vi "ASIOInfo.vi"() -> ()   [LabVIEW 2016]
uses:
  WaveIO.llb/ASIO_Informations.ctl
panel:
  out "ASIO Device Infos":T1[](array[typedef])
  in  "Direction (Input)":u16(ring)=3 items=["Input", "Output", "Loopback", "ASIO input", "ASIO output"]
  out "Number of Devices":i32=1
  # "ASIO is a trademark and software of \nSteinberg Media Technologies GmbH"
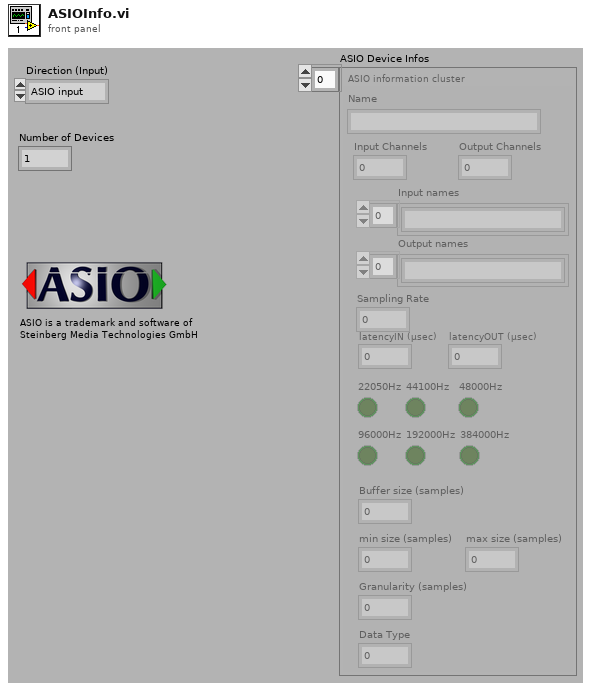
[diagram p1: front panel]
types:
  T1 = typedef "ASIO_Informations.ctl" = cluster{"Input Channels":i32, "Output Channels":i32, "Sampling Rate":i32, "22050Hz":bool, "44100Hz":bool, "48000Hz":bool, "96000Hz":bool, "192000Hz":bool, "Buffer size (samples)":i32, "min size (samples)":i32, "max size (samples)":i32, "Granularity (samples)":i32, "Name":string, "Data Type":i32, "latencyIN (µsec)":i32, "latencyOUT (µsec)":i32, "Input names":string[], "Output names":string[], "384000Hz":bool}
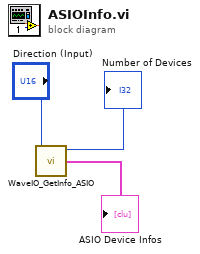
[diagram p0: block diagram]
diagram:
  n1 = call "WaveIO_GetInfo_ASIO.vi"("Direction (Input)"="Direction (Input)") -> ("numdev"=→"Number of Devices":i32, "ASIO Device Infos"=→"ASIO Device Infos":T1[])  [unwired: 3 out]
